vi "Acquisition.vi"() -> ()   [LabVIEW 2016]
uses:
  MainFGV/MainFGV_mods.ctl
  Log/log_mods.ctl
  Tools/variable_acess_mods.ctl
  Tools/main_display_modes.ctl
panel:
  in  "leave":bool
  in  "advanced":bool
  in  "settings":bool
  in  "stop":bool
  in  "reset":bool
  in  "start":bool
  in  "tab":T1(tab)
  out "RMSacel":dbl[][](graph) caption="Acelerômetros"
  out "RMShammer":dbl(graph) caption="Martelo"
  out "Nyquist":cluster{dbl[], dbl[]}[](graph) caption="XY Graph"
  out "inert":waveform(dbl)[](graph) caption="Inertância"
  out "acelTime":waveform(dbl)[](graph) caption="Acelerômetros - Sinal no tempo"
  out "hammerSpec":waveform(dbl)(graph) caption="Martelo - Espectro"
  out "hammerTime":waveform(dbl)(graph) caption="Martelo - Sinal no tempo"
  out "meanInert":waveform(dbl)[](graph) caption="Inertância média"
  out "progress":dbl(slide)=1.0 caption="Inativo" scale=0.0..1.0
  in  "active":bool
  in  "TestName":string caption="Nome do ensaio"
  in  "TestDir":path=path "C:/Users/l01481/Desktop/nada" caption="Diretório do ensaio"
  in  "Log":string
  # "Análise modal\n\nAquisição\n\nLink do repositório: https://github.com/LeonardoSirino/ModalAnalysis"
  # "Leonardo Sirino\nSistemas Mecânicos \nT + 55 (41) 3361-6152 | C + 55 (41) 99679-007\nleonardo.sirino@lactec.org.br | www.lactec.org.br"
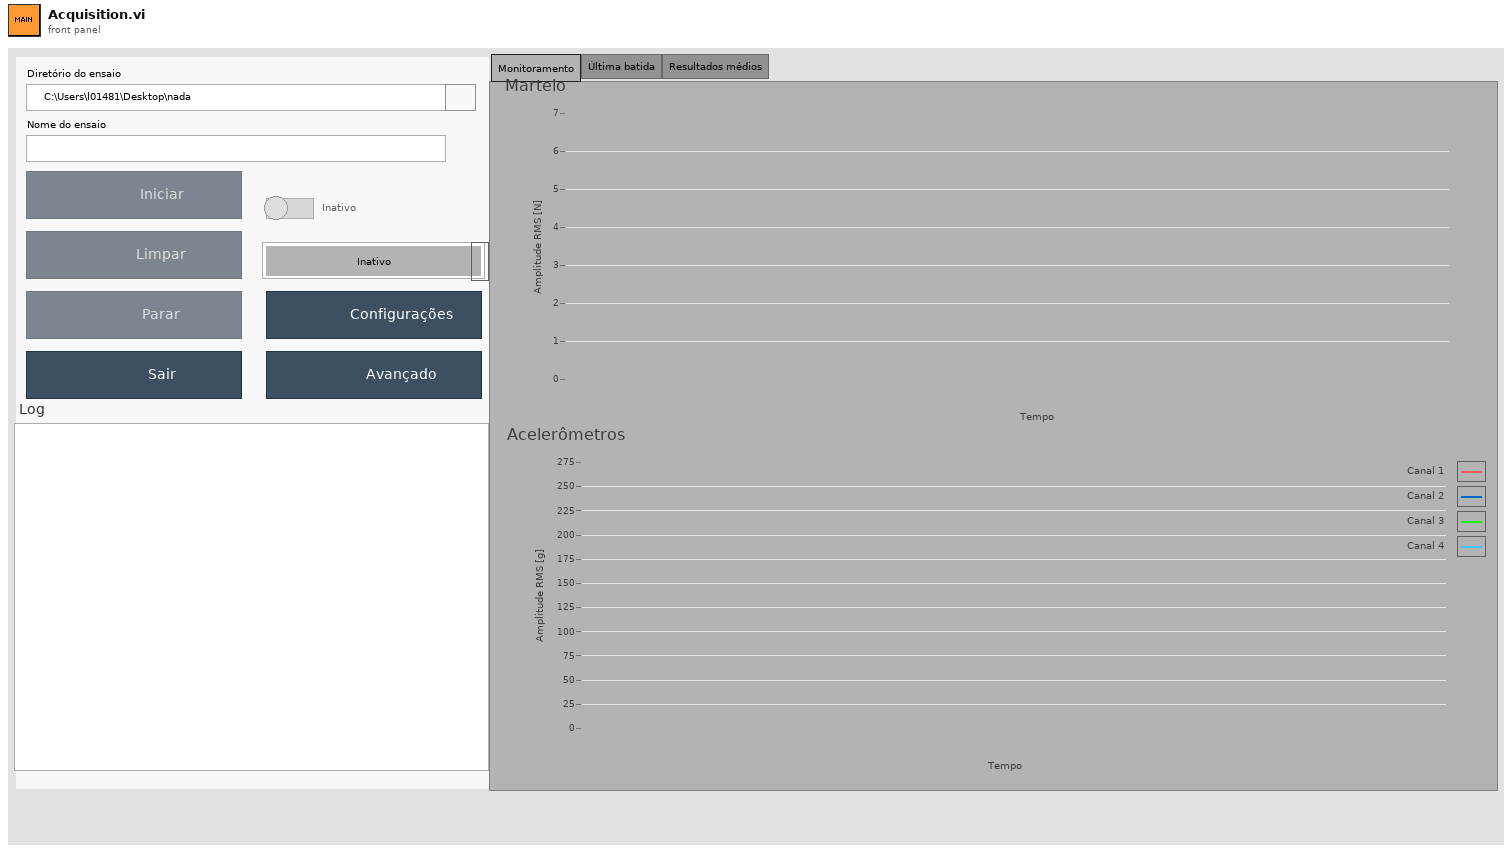
[diagram p1: front panel]
types:
  T1 = enum32{"Monitoramento", "Última batida", "Resultados médios"}
  T2 = typedef "log_mods.ctl" = enum16{"Init", "SetStatus", "RMSacel", "HitData", "Clear", "PeakForce", "WriteToLog", "End"}
  T3 = typedef "MainFGV_mods.ctl" = enum16{"Init", "Config", "Advanced", "CreateTask", "Register", "Start", "Record", "End"}
  T4 = typedef "main_display_modes.ctl" = enum16{"init", "after_config", "after_start", "end"}
  T5 = typedef "variable_acess_mods.ctl" = enum16{"init", "set", "get"}
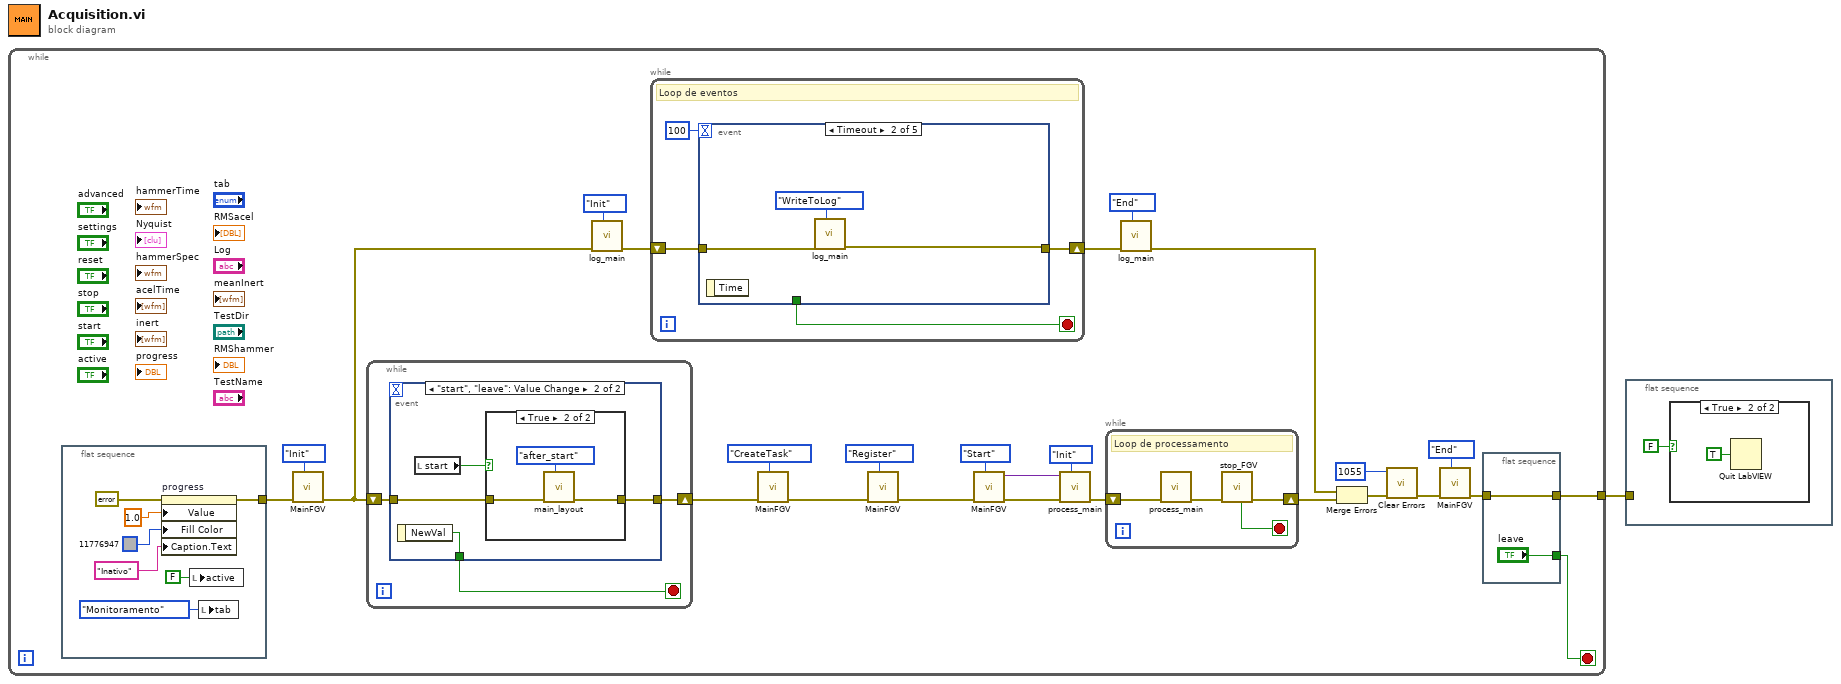
[diagram p0: block diagram]
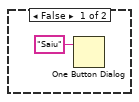
[diagram p2: hidden frame]
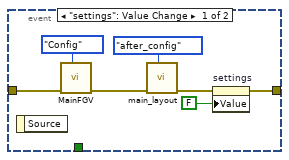
[diagram p3: hidden frame]
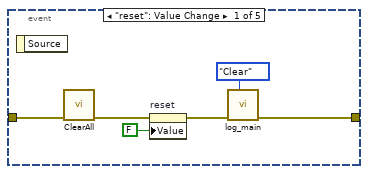
[diagram p5: hidden frame]
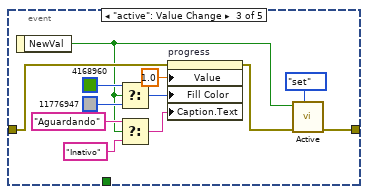
[diagram p6: hidden frame]
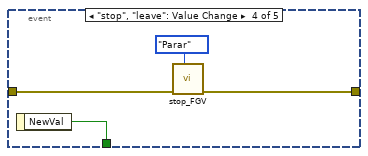
[diagram p7: hidden frame]
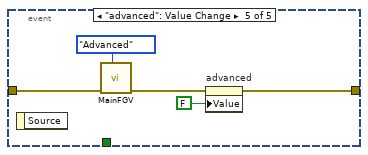
[diagram p8: hidden frame]
diagram:
  n1 = while {
    tunnel: [w4] -> w1
    stop <- w2 stop-if-true
    n2 = flat-sequence {
      tunnel: [w33] -> w7
      frame #0 {
        n3 = property on="progress" class="Slide (strict)"(error in=errorcluster {"status"=FALSE, "code"=0, "source"=""} ("Error In"), "Value"=1.0 ("progress"), "Fill Color"=u32 11776947, "Caption.Text"="Inativo") -> (error out=w33:errorcluster)  [unwired: 1 in, 1 out]
        n4 = local write "active"(FALSE ("active")) -> ()
        n5 = local write "tab"(T1."Monitoramento" ("tab")) -> ()
      }
    }
    n6 = call "MainFGV.vi"("FGV_mods"=MainFGV_mods."Init", "Error In"=w7) -> ("Error Out"=w14:errorcluster)  [unwired: 8 in, 1 out]
    n7 = while {
      shift-right: [w38] -> w25
      shift-left: w14 -> [w39]
      stop <- w37 stop-if-true
      n8 = event shown="[1] \"start\", \"leave\": Value Change" {
        selector: _ -> [_ _]
        dyn-events: _ -> [_ _]
        timeout: _ -> [_ _]
        tunnel: w39 -> [w45 w48]
        tunnel: [w44 w47] -> w38
        tunnel: [_ w50] -> w37
        event "settings": Value Change {
          n9 = event-data() -> ()  [unwired: 1 in, 1 out]
          n10 = call "MainFGV.vi"("FGV_mods"=MainFGV_mods."Config", "Error In"=w45) -> ("Error Out"=w41:errorcluster)  [unwired: 8 in, 1 out]
          n11 = call "main_layout.vi"("layout_mode"=main_display_modes."after_config", "error in"=w41) -> ("error out"=w40:errorcluster)  [unwired: 9 in]
          n12 = property on="settings" class="Bool (strict)"(error in=w40, "Value"=FALSE ("config")) -> (error out=w44:errorcluster)  [unwired: 1 in, 1 out]
        }
        event "start", "leave": Value Change {
          n13 = event-data() -> ("NewVal"=w50:bool)  [unwired: 1 in]
          n14 = local read "start"() -> (w49:bool)
          n15 = case shown="True" w49 {
            tunnel: w48 -> [w51 w53]
            tunnel: [w51 w52] -> w47
            frame False {
            }
            frame True {
              n16 = call "main_layout.vi"("layout_mode"=main_display_modes."after_start", "error in"=w53) -> ("error out"=w52:errorcluster)  [unwired: 9 in]
            }
          }
        }
      }
    }
    n17 = call "log_main.vi"("FGV_mods"=log_mods."Init", "Error In"=w14) -> ("Error Out"=w8:errorcluster)  [unwired: 9 in]
    n18 = while {
      shift-right: [w57] -> w10
      shift-left: w8 -> [w58]
      stop <- w56 stop-if-true
      # "Loop de eventos"
      n19 = event shown="[1] Timeout" {
        selector: _ -> [_ _ _ _ _]
        dyn-events: _ -> [_ _ _ _ _]
        timeout: 100 -> [_ _ _ _ _]
        tunnel: w58 -> [w64 w66 w78 w82 w87]
        tunnel: [w62 w65 w69 w81 w85] -> w57
        tunnel: [_ _ _ w83 _] -> w56
        event "reset": Value Change {
          n20 = event-data() -> ()  [unwired: 1 in, 1 out]
          n21 = call "ClearAll.vi"("error in"=w64) -> ("error out"=w61:errorcluster)  [unwired: 10 in]
          n22 = property on="reset" class="Bool (strict)"(error in=w61, "Value"=FALSE ("clear")) -> (error out=w60:errorcluster)  [unwired: 1 in, 1 out]
          n23 = call "log_main.vi"("FGV_mods"=log_mods."Clear", "Error In"=w60) -> ("Error Out"=w62:errorcluster)  [unwired: 9 in]
        }
        event Timeout {
          n24 = event-data() -> ()  [unwired: 1 in, 1 out]
          n25 = call "log_main.vi"("FGV_mods"=log_mods."WriteToLog", "Error In"=w66) -> ("Error Out"=w65:errorcluster)  [unwired: 9 in]
        }
        event "active": Value Change {
          n26 = event-data() -> ("NewVal"=w68:bool)  [unwired: 1 in]
          n27 = Select(t=u32 4168960, s=w68, f=u32 11776947) -> (s? t:f=w75:u32)
          n28 = Select(t="Aguardando", s=w68, f="Inativo") -> (s? t:f=w74:string)
          n29 = property on="progress" class="Slide (strict)"(error in=w78, "Value"=1.0 ("progress"), "Fill Color"=w75, "Caption.Text"=w74) -> (error out=w70:errorcluster)  [unwired: 1 in, 1 out]
          n30 = call "Active.vi"("FGV_mods"=variable_acess_mods."set", "Error In"=w70, "value"=w68) -> ("Error Out"=w69:errorcluster)  [unwired: 7 in, 1 out]
        }
        event "stop", "leave": Value Change {
          n31 = event-data() -> ("NewVal"=w83:bool)  [unwired: 1 in]
          n32 = call "stop_FGV.vi"("comandos"=enum16{"Iniciar", "Parar", "Parar?"}."Parar", "error in (no error)"=w82) -> ("error out"=w81:errorcluster)  [unwired: 8 in, 1 out]
        }
        event "advanced": Value Change {
          n33 = event-data() -> ()  [unwired: 1 in, 1 out]
          n34 = call "MainFGV.vi"("FGV_mods"=MainFGV_mods."Advanced", "Error In"=w87) -> ("Error Out"=w86:errorcluster)  [unwired: 8 in, 1 out]
          n35 = property on="advanced" class="Bool (strict)"(error in=w86, "Value"=FALSE ("config")) -> (error out=w85:errorcluster)  [unwired: 1 in, 1 out]
        }
      }
    }
    n36 = call "MainFGV.vi"("FGV_mods"=MainFGV_mods."CreateTask", "Error In"=w25) -> ("Error Out"=w23:errorcluster)  [unwired: 8 in, 1 out]
    n37 = call "MainFGV.vi"("FGV_mods"=MainFGV_mods."Register", "Error In"=w23) -> ("Error Out"=w21:errorcluster)  [unwired: 8 in, 1 out]
    n38 = call "MainFGV.vi"("FGV_mods"=MainFGV_mods."Start", "Error In"=w21) -> ("Error Out"=w12:errorcluster, "DataOut"=w16:variant)  [unwired: 8 in]
    n39 = call "process_main.vi"("FGV_mods"=enum16{"Init", "Exec", "End"}."Init", "Error In"=w12, "DataIn"=w16) -> ("Error Out"=w15:errorcluster)  [unwired: 8 in]
    n40 = while {
      shift-right: [w90] -> w19
      shift-left: w15 -> [w92]
      stop <- w89 stop-if-true
      # "Loop de processamento"
      n41 = call "process_main.vi"("Error In"=w92) -> ("Error Out"=w91:errorcluster)  [unwired: 10 in]
      n42 = call "stop_FGV.vi"("error in (no error)"=w91) -> ("error out"=w90:errorcluster, "parar?"=w89:bool)  [unwired: 9 in]
    }
    n43 = call "log_main.vi"("FGV_mods"=log_mods."End", "Error In"=w10) -> ("Error Out"=w9:errorcluster)  [unwired: 9 in]
    n44 = Merge Errors(w9, w19) -> (w18:errorcluster)
    n45 = call <vilib>:"Clear Errors.vi"("error in (no error)"=w18, "specific error code to clear (0: all)"=1055) -> ("error out"=w6:errorcluster)  [unwired: 4 in, 1 out]
    n46 = call "MainFGV.vi"("FGV_mods"=MainFGV_mods."End", "Error In"=w6) -> ("Error Out"=w3:errorcluster)  [unwired: 8 in, 1 out]
    n47 = flat-sequence {
      tunnel: [w29] -> w4
      tunnel: w3 -> [w29]
      tunnel: ["leave"] -> w2
      frame #0 {
      }
    }
  }
  n48 = flat-sequence {
    tunnel: w1 -> [_]
    frame #0 {
      n49 = case shown="True" FALSE {
        frame False {
          n50 = One Button Dialog(message="Saiu") -> ()  [unwired: 1 in, 1 out]
        }
        frame True {
          n51 = Quit LabVIEW(quit? (T)=TRUE) -> ()
        }
      }
    }
  }
